vi "AlazarSetClockSwitchOver.vi"(3 "error in (no error)":errorcluster, 4 "DummyClockOnTime_ns":u32, 5 "Mode":u32(ring) items=["Disable", "Enable"], 6 "Handle":u64) -> (0 "error out":errorcluster, 1 "Return Code":u32, 2 "Handle":u64)   [LabVIEW 2018]
doc: "Configure the dummy clock.\n\nWhen the \"dummy clock\" option enabled, the digitizer uses an internally generated clock signal to drive its ADCs for a specified amount of time after the end of each record. At the end of the dummy clock on time, the digitizer switches back to using the external clock signal to clock the ADCs.\n\nScanning applications that generate an unusable external clock signal during horizontal retrace periods at the end of each scan line should consider enabling the \"dummy clock\" option."
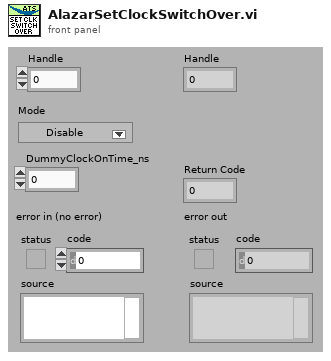
[diagram p1: front panel]
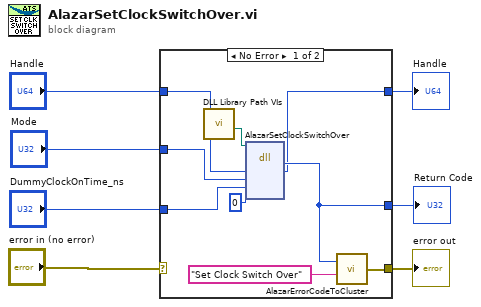
[diagram p0: block diagram]
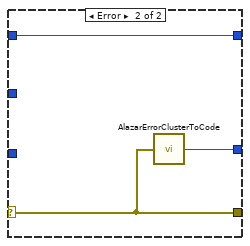
[diagram p2: hidden frame]
diagram:
  n1 = case shown="No Error" "error in (no error)" {
    selector: "error in (no error)" -> [_ w19]
    tunnel: [w13 w19] -> w6
    tunnel: [w15 w18] -> w5
    tunnel: "Handle" -> [w16 w17]
    tunnel: [w12 w17] -> w3
    tunnel: "Mode" -> [w11 _]
    tunnel: "DummyClockOnTime_ns" -> [w10 _]
    frame No Error {
      n2 = call "DLL Library Path VIs.vi"() -> ("Alazar"=w8:path)  [unwired: 9 in, 2 out]
      n3 = dll-call lib="C:/Project/SerialSectOCT - FFT GPU/SerialSectOCT/Labview Software/DLL/ATSApi.dll" fn="AlazarSetClockSwitchOver"(path in=w8, "handle"=w16, "mode"=w11, "dummyClockOnTime_ns"=w10, "reserved"=u32 0) -> ("return type"=w15:u32, "handle"=w12:u64)  [unwired: 5 in, 2 out]
      n4 = call "AlazarErrorCodeToCluster.vi"("Message"="Set Clock Switch Over", "Error Code"=w15) -> ("error out"=w13:errorcluster)
    }
    frame Error {
      n5 = call "AlazarErrorClusterToCode.vi"("error in (no error)"=w19) -> ("Error Code"=w18:u32)
    }
  }
  "Handle" <- w3
  "error out" <- w6
  "Return Code" <- w5
